vi "USBImageContinuousV1.5.vi"() -> ()   [LabVIEW 2017]
uses:
  <vilib>/Utility/file.llb/Write Delimited Spreadsheet (I64).vi
  atmcd32d.dll
panel:
  in  "Tab Control":T1(tab)
  out "Expected position on spectrometer (pixels):":dbl
  in  "Harmonic":dbl min=10.0 max=40.0
  out "l (nm)":dbl
  out "E (J)":dbl
  out "E (eV)":dbl
  out "Nearest Harmonic of 800nm":dbl
  out "Cursor Position (pixels)":dbl
  out "Distance to nearest harmonic of 800nm (pixels)":dbl
  in  "Grating:":u16(ring) items=["Shimadzu 30-006  "]
  in  "Laser:":u16(ring) items=["800nm  "]
  in  "Trigger":u32(ring) items=["Internal", "External"]
  in  "Exposure Time (secs)":sgl format="%.2f"
  out "Get Acquired Data":u32
  out "Start Acquisition":u32
  out "Detector X Pixels":i32
  out "Detector Y Pixels":i32
  out "Shut Down":u32
  out "Raw Image":i32[][](graph)
  out "Vertical Binned image":i32[](graph)
  out "Get Status":u32
  in  "Stop":bool
  in  "?":bool
  out "Camera Status:":bool
  out "Last Image Saved:":string
  in  "Calibration Date":u16(ring) items=["first calibration - 7/31", "7/31-current"]
  out "Calibration Date: indicator:":u16(ring) items=["first calibration - 7/31", "7/31-current"]
  out "Status":u32
  out "Camera outputs":T2
  out "Camera inputs":T3
  out "Wavelength Graph (nm)":cluster{"No prefix":dbl, i32}[](graph)
  out "Energy Graph (eV)":cluster{"eV":dbl, i32}[](graph)
  out "Harmonics Graph":cluster{"No prefix":dbl, i32}[](graph)
  # "Acquisition Mode: Single Scan\nReadout Mode: Full Resolution Image"
  # "Return values"
  # "XUV Spectrometer Control VI"
  # "Status"
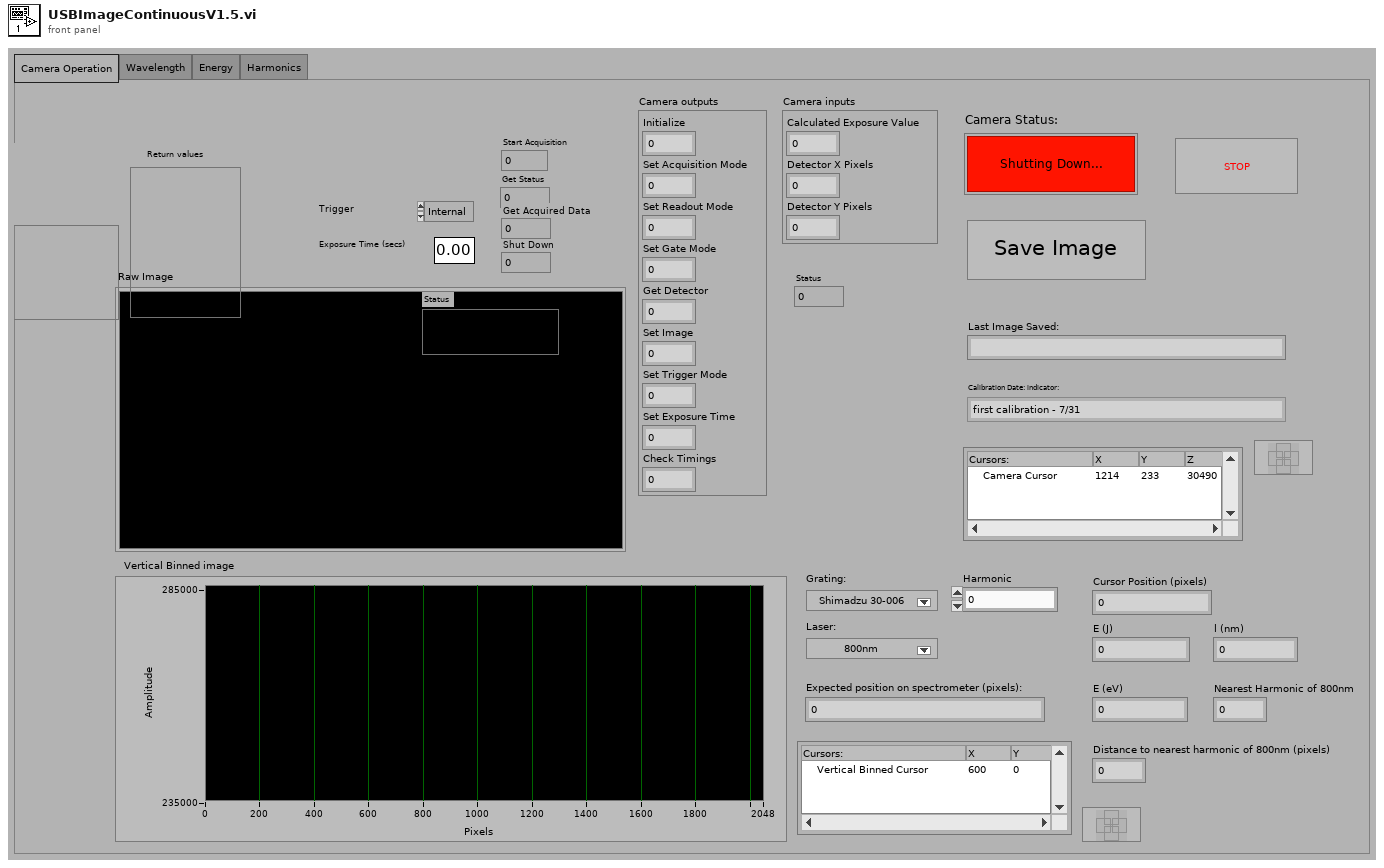
[diagram p1: front panel]
types:
  T1 = enum32{"Camera Operation", "Wavelength", "Energy", "Harmonics"}
  T2 = cluster{"Initialize":u32, "Set Acquisition Mode":u32, "Set Readout Mode":u32, "Set Gate Mode":u32, "Get Detector":u32, "Set Image":u32, "Set Trigger Mode":u32, "Set Exposure Time":u32, "Check Timings":u32}
  T3 = cluster{"Calculated Exposure Value":sgl, "Detector X Pixels":i32, "Detector Y Pixels":i32}
  T4 = cluster{"DRV_SUCCESS":i32, "to shutdown":bool, "to get acquired data":bool, "to start acquisition":bool}
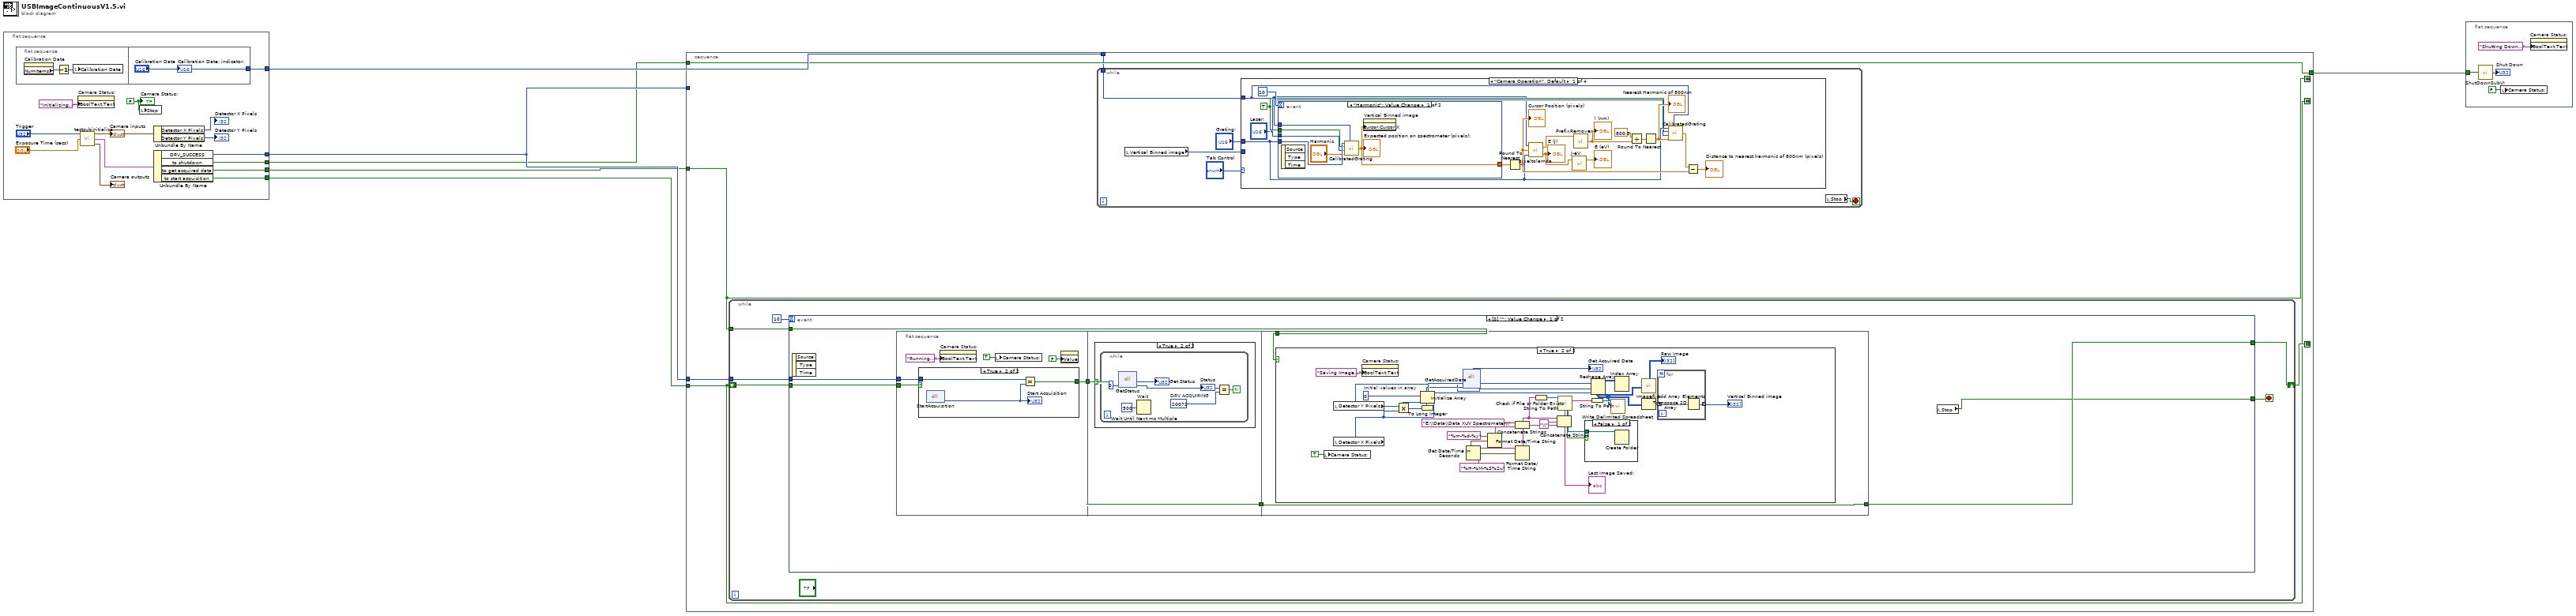
[diagram p0: block diagram]
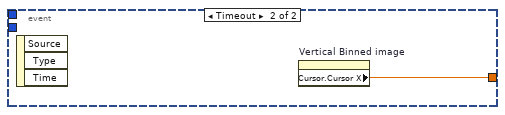
[diagram p2: hidden frame]
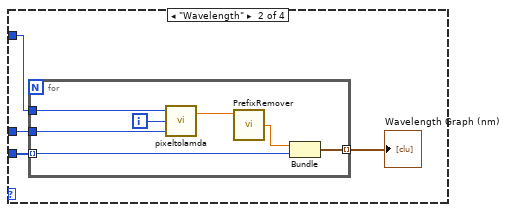
[diagram p3: hidden frame]
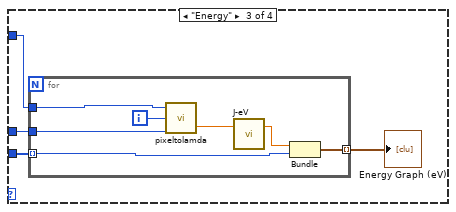
[diagram p4: hidden frame]
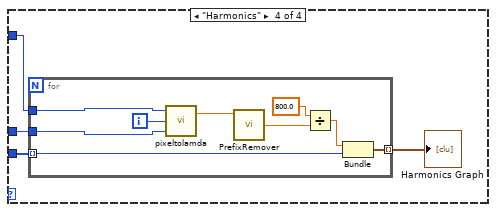
[diagram p5: hidden frame]
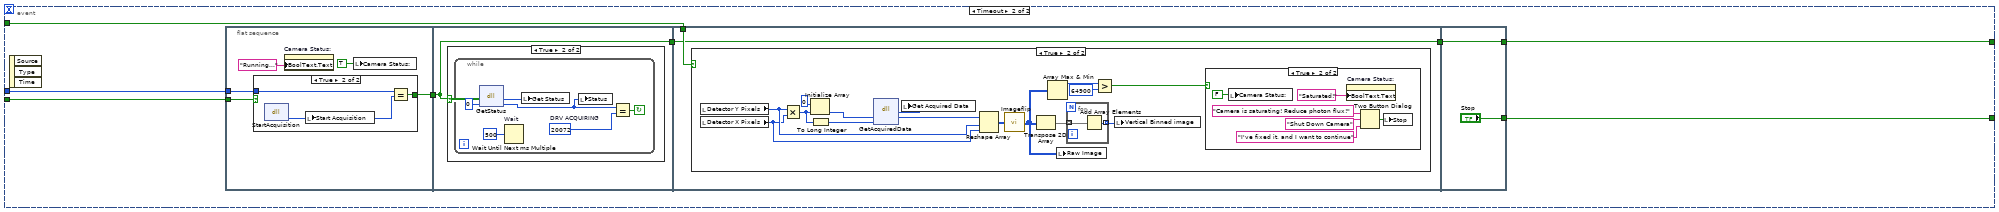
[diagram p10: hidden frame]
diagram:
  n1 = flat-sequence {
    tunnel: [w7] -> w6
    tunnel: [w8] -> w5
    tunnel: [w9] -> w4
    tunnel: [w10] -> w1
    tunnel: [w17] -> w2
    frame #0 {
      w18 = FALSE ("Camera Status:")
      n2 = flat-sequence {
        tunnel: ["Calibration Date"] -> w17
        frame #0 {
          n3 = property on="Calibration Date" class="Ring (strict)"() -> ("NumItems"=w22:u32)  [unwired: 2 in, 2 out]
          n4 = Decrement(x=w22) -> (x-1=w21:u32)
          n5 = local write "Calibration Date"(w21) -> ()
        }
        frame #1 {
          "Calibration Date: indicator:" <- "Calibration Date"
        }
      }
      n6 = property on="Camera Status:" class="Bool (strict)"("BoolText.Text"="Initializing..." ("String")) -> ()  [unwired: 2 in, 2 out]
      n7 = call "testsubinitialize.vi"("Exposure Time (secs)"="Exposure Time (secs)", "Trigger"="Trigger") -> ("Camera outputs"=→"Camera outputs":T2, "Camera status"=w14:T4, "Camera inputs"=w13:T3)  [unwired: 1 in]
      "Camera inputs" <- w13
      n8 = local write "Stop"(w18) -> ()
      n9 = Unbundle By Name(w13) -> ("Detector X Pixels"=→"Detector X Pixels":i32, "Detector Y Pixels"=→"Detector Y Pixels":i32)
      n10 = Unbundle By Name(w14) -> ("DRV_SUCCESS"=w7:i32, "to shutdown"=w10:bool, "to get acquired data"=w9:bool, "to start acquisition"=w8:bool)
      "Camera Status:" <- w18
    }
  }
  n11 = stacked-sequence {
    seq-local: [w27] -> [_]
    seq-local: [w28] -> [_]
    seq-local: [w26] -> [_]
    tunnel: w6 -> [_]
    tunnel: w6 -> [w29]
    tunnel: w5 -> [w27]
    tunnel: w4 -> [w26]
    tunnel: w1 -> [w25]
    tunnel: [w25] -> w3
    tunnel: w2 -> [w24]
    frame #0 {
      n12 = while {
        tunnel: w29 -> [w97]
        tunnel: w26 -> [w95]
        shift-right: [w96] -> w28
        shift-left: w27 -> [w98]
        stop <- w93 stop-if-true
        n13 = event shown="[0] \"\": Value Change" {
          selector: _ -> [_ _]
          dyn-events: _ -> [_ _]
          timeout: 10 -> [_ _]
          tunnel: w98 -> [w103 w160]
          tunnel: w97 -> [w102 w159]
          tunnel: [w101 w158] -> w96
          tunnel: w95 -> [w100 w157]
          tunnel: [w99 w156] -> w93
          event Value Change {
            n14 = event-data() -> ()  [unwired: 1 in, 3 out]
            n15 = flat-sequence {
              tunnel: w103 -> [w111]
              tunnel: w102 -> [w110]
              tunnel: [w109] -> w105
              tunnel: w105 -> [w116]
              tunnel: [w116] -> w104
              tunnel: [w124] -> w101
              tunnel: w104 -> [w124]
              tunnel: w100 -> [w123]
              frame #0 {
                n16 = case shown="True" w111 {
                  tunnel: [FALSE w114] -> w109
                  tunnel: w110 -> [_ w113]
                  frame False {
                  }
                  frame True {
                    n17 = dll-call lib="atmcd32d.dll" fn="StartAcquisition" label="Call Library Function start acquisition"() -> (w115:u32)  [unwired: 3 in, 2 out]
                    "Start Acquisition" <- w115
                    n18 = Equal?(x=w113, y=w115) -> (x = y?=w114:bool)
                  }
                }
                n19 = property on="Camera Status:" class="Bool (strict)"("BoolText.Text"="Running..." ("Boolean Text.Text")) -> ()  [unwired: 2 in, 2 out]
                n20 = local write "Camera Status:"(TRUE ("Camera Status:")) -> ()
                n21 = property class="Bool (strict)"("Value"=FALSE ("Take image")) -> ()  [unwired: 2 in, 2 out]
              }
              frame #1 {
                n22 = case shown="True" w116 {
                  frame False {
                  }
                  frame True {
                    n23 = while {
                      stop <- w120 continue-if-true
                      w119 = u16 20072  # DRV ACQUIRING
                      n24 = dll-call lib="atmcd32d.dll" fn="GetStatus" label="Call Library Function GetAcquisitionStatus"(u16 0) -> (→"Get Status":u32, w118:u32)  [unwired: 3 in, 2 out]
                      "Status" <- w118
                      n25 = Wait Until Next ms Multiple "Wait"(millisecond multiple=u32 500) -> ()  [unwired: 1 out]
                      n26 = Equal?(x=w118, y=w119) -> (x = y?=w120:bool)
                    }
                  }
                }
              }
              frame #2 {
                n27 = case shown="True" w123 {
                  frame False {
                  }
                  frame True {
                    w151 = 0  # Initial values in array
                    n28 = local write "Camera Status:"(TRUE ("Camera Status:")) -> ()
                    n29 = local read "Detector Y Pixels"() -> (w145:i32)
                    n30 = local read "Detector X Pixels"() -> (w144:i32)
                    n31 = property on="Camera Status:" class="Bool (strict)"("BoolText.Text"="Saving Image..." ("Boolean Text.Text")) -> ()  [unwired: 2 in, 2 out]
                    n32 = Multiply(x=w145, y=w144) -> (x*y=w147:i32)
                    n33 = To Long Integer(number=w147) -> (32bit integer=w148:i32)
                    n34 = Initialize Array "Initialize Array"(w151, w147) -> (w149:i32[])
                    n35 = dll-call lib="atmcd32d.dll" fn="GetAcquiredData" label="Call Library Function Get Acquired data"(w149, w148) -> (→"Get Acquired Data":u32, w146:i32[])  [unwired: 4 in, 2 out]
                    n36 = Get Date/Time In Seconds() -> (seconds since 1Jan1904=w141:timestamp)
                    n37 = Format Date/Time String(time format string (%c)="%m-%d-%y", seconds (now)=w141) -> (date/time string=w139:string)  [unwired: 1 in]
                    n38 = Concatenate Strings("E:\\Data\\Data XUV Spectrometer\\" ("string"), w139) -> (w142:string)
                    n39 = Format Date/Time String(time format string (%c)="%H-%M-%S%2u", seconds (now)=w141) -> (date/time string=w140:string)  [unwired: 1 in]
                    n40 = String To Path(string=w142) -> (path=w138:path)
                    n41 = Concatenate Strings(w142, "\\" ("string"), w140) -> (w143:string)
                    "Last Image Saved:" <- w143
                    n42 = call <vilib>:"Check if File or Folder Exists.vi"("path"=w138) -> ("file or folder exists?"=w136:bool, "dup path"=w137:path)  [unwired: 8 in, 1 out]
                    n43 = case shown="False" w136 {
                      tunnel: w137 -> [w154 _]
                      frame False {
                        n44 = Create Folder(path (use dialog)=w154) -> ()  [unwired: 2 in, 3 out]
                      }
                      frame True {
                      }
                    }
                    n45 = String To Path(string=w143) -> (path=w131:path)
                    n46 = Reshape Array(w146, w145, w144) -> (w126:i32[][])
                    n47 = call-poly <vilib>:"Write Delimited Spreadsheet.vi"("file path (dialog if empty)"=w131, "2D data"=w126) -> ()  [unwired: 12 in, 2 out]
                    n48 = Index Array(array=w126) -> ()  [unwired: 2 in, 1 out]
                    n49 = call "Imageflip.vi"("2D array"=w126) -> ("transposed array"=→"Raw Image":i32[][])
                    n50 = Transpose 2D Array(2D array=w126) -> (transposed array=w130:i32[][])
                    n51 = for {
                      tunnel: w130 -> [w153] mode=indexing
                      tunnel: [w152] -> w129 mode=indexing
                      n52 = Add Array Elements(numeric array=w153) -> (sum=w152:i32)
                    }
                    "Vertical Binned image" <- w129
                  }
                }
              }
            }
            n53 = local read "Stop"() -> (w99:bool)
          }
          event Timeout {
            n54 = event-data() -> ()  [unwired: 1 in, 3 out]
            n55 = flat-sequence {
              tunnel: w160 -> [w167]
              tunnel: w159 -> [w166]
              tunnel: [w165] -> w162
              tunnel: w162 -> [w172]
              tunnel: [w172] -> w161
              tunnel: w161 -> [w179]
              tunnel: w157 -> [w180]
              tunnel: [w179] -> w155
              tunnel: [w205] -> w158
              tunnel: w155 -> [w205]
              tunnel: ["Stop"] -> w156
              frame #0 {
                n56 = case shown="True" w167 {
                  tunnel: [FALSE w171] -> w165
                  tunnel: w166 -> [_ w170]
                  frame False {
                  }
                  frame True {
                    n57 = dll-call lib="atmcd32d.dll" fn="StartAcquisition" label="Call Library Function start acquisition"() -> (w169:u32)  [unwired: 3 in, 2 out]
                    n58 = local write "Start Acquisition"(w169) -> ()
                    n59 = Equal?(x=w170, y=w169) -> (x = y?=w171:bool)
                  }
                }
                n60 = property on="Camera Status:" class="Bool (strict)"("BoolText.Text"="Running..." ("Boolean Text.Text")) -> ()  [unwired: 2 in, 2 out]
                n61 = local write "Camera Status:"(TRUE ("Camera Status:")) -> ()
              }
              frame #1 {
                n62 = case shown="True" w172 {
                  frame False {
                  }
                  frame True {
                    n63 = while {
                      stop <- w176 continue-if-true
                      w175 = u16 20072  # DRV ACQUIRING
                      n64 = dll-call lib="atmcd32d.dll" fn="GetStatus" label="Call Library Function GetAcquisitionStatus"(u16 0) -> (w174:u32, w173:u32)  [unwired: 3 in, 2 out]
                      n65 = Wait Until Next ms Multiple "Wait"(millisecond multiple=u32 500) -> ()  [unwired: 1 out]
                      n66 = local write "Get Status"(w174) -> ()
                      n67 = local write "Status"(w173) -> ()
                      n68 = Equal?(x=w173, y=w175) -> (x = y?=w176:bool)
                    }
                  }
                }
              }
              frame #2 {
                n69 = case shown="True" w180 {
                  frame False {
                  }
                  frame True {
                    n70 = local read "Detector Y Pixels"() -> (w190:i32)
                    n71 = local read "Detector X Pixels"() -> (w183:i32)
                    n72 = Multiply(x=w190, y=w183) -> (x*y=w192:i32)
                    n73 = Initialize Array "Initialize Array"(0 ("Initial values in array"), w192) -> (w194:i32[])
                    n74 = To Long Integer(number=w192) -> (32bit integer=w193:i32)
                    n75 = dll-call lib="atmcd32d.dll" fn="GetAcquiredData" label="Call Library Function Get Acquired data"(w194, w193) -> (w188:u32, w191:i32[])  [unwired: 4 in, 2 out]
                    n76 = local write "Get Acquired Data"(w188) -> ()
                    n77 = Reshape Array(w191, w190, w183) -> (w181:i32[][])
                    n78 = call "Imageflip.vi"("2D array"=w181) -> ("transposed array"=w182:i32[][])
                    n79 = Transpose 2D Array(2D array=w182) -> (transposed array=w189:i32[][])
                    n80 = Array Max & Min(array=w182) -> (max value=w186:i32)  [unwired: 3 out]
                    n81 = local write "Raw Image"(w182) -> ()
                    n82 = for {
                      tunnel: w189 -> [w203] mode=indexing
                      tunnel: [w202] -> w187 mode=indexing
                      n83 = Add Array Elements(numeric array=w203) -> (sum=w202:i32)
                    }
                    n84 = Greater?(x=w186, y=64900) -> (0:w184:bool)
                    n85 = local write "Vertical Binned image"(w187) -> ()
                    n86 = case shown="True" w184 {
                      frame False {
                      }
                      frame True {
                        n87 = local write "Camera Status:"(FALSE ("Camera Status:")) -> ()
                        n88 = property on="Camera Status:" class="Bool (strict)"("BoolText.Text"="Saturated!" ("Boolean Text.Text")) -> ()  [unwired: 2 in, 2 out]
                        n89 = Two Button Dialog(message="Camera is saturating! Reduce photon flux!", 1:"I've fixed it, and I want to continue" ("message"), 2:"Shut Down Camera" ("T button name (\"OK\")")) -> (T button?=w197:bool)
                        n90 = local write "Stop"(w197) -> ()
                      }
                    }
                  }
                }
              }
              frame #3 {
              }
            }
          }
        }
      }
      n91 = while {
        tunnel: w24 -> [w30]
        stop <- w31 stop-if-true
        n92 = local read "Vertical Binned image"() -> (w33:i32[])
        n93 = case shown="\"Camera Operation\", Default" "Tab Control" {
          tunnel: w33 -> [_ w61 w72 w83]
          tunnel: "Grating:" -> [w38 w60 w71 w82]
          tunnel: w30 -> [w35 w58 w69 w80]
          frame "Camera Operation", Default {
            w37 = TRUE
            n94 = event shown="[0] \"Harmonic\": Value Change" {
              selector: _ -> [_ _]
              dyn-events: _ -> [_ _]
              timeout: 10 -> [_ _]
              tunnel: [w52 w57] -> w39
              tunnel: w38 -> [w56 _]
              tunnel: w37 -> [w55 _]
              tunnel: "Laser:" -> [w54 _]
              tunnel: w35 -> [w53 _]
              event "Harmonic": Value Change {
                n95 = event-data() -> ()  [unwired: 1 in, 3 out]
                n96 = call "CalibratedGrating.vi"("Grating:"=w56, "Subvi?"=w55, "Laser:"=w54, "Harmonic"="Harmonic", "Caibration Date"=w53) -> ("Position on spectrometer (pixels):"=w52:dbl)
                "Expected position on spectrometer (pixels):" <- w52
                n97 = property on="Vertical Binned image" class="WFGraph (strict)"("Cursor.Cursor X"=w52) -> ()  [unwired: 2 in, 2 out]
              }
              event Timeout {
                n98 = event-data() -> ()  [unwired: 1 in, 3 out]
                n99 = property on="Vertical Binned image" class="WFGraph (strict)"() -> ("Cursor.Cursor X"=w57:dbl)  [unwired: 2 in, 2 out]
              }
            }
            n100 = Round To Nearest(number=w39) -> (nearest integer value=w44:dbl)
            "Cursor Position (pixels)" <- w44
            n101 = call "pixeltolamda.vi"("Grating:"=w38, "Pixel Postion"=w44, "Caibration Date"=w35) -> ("E (J)"=w46:dbl, "lamda (m)"=w50:dbl)
            "E (J)" <- w46
            n102 = call "J-eV.vi"("J"=w46) -> ("eV"=→"E (eV)":dbl)  [unwired: 1 in, 1 out]
            n103 = call "PrefixRemover.vi"("Nano"=w50) -> ("No prefix"=w47:dbl)  [unwired: 3 in]
            "l (nm)" <- w47
            n104 = Divide(x=800.0, y=w47) -> (x/y=w49:dbl)
            n105 = Round To Nearest(number=w49) -> (nearest integer value=w43:dbl)
            "Nearest Harmonic of 800nm" <- w43
            n106 = call "CalibratedGrating.vi"("Grating:"=w38, "Subvi?"=w37, "Laser:"="Laser:", "Harmonic"=w43, "Caibration Date"=w35) -> ("Position on spectrometer (pixels):"=w42:dbl)
            n107 = Subtract(x=w42, y=w44) -> (x-y=→"Distance to nearest harmonic of 800nm (pixels)":dbl)
          }
          frame "Wavelength" {
            n108 = for {
              tunnel: w61 -> [w64] mode=indexing
              tunnel: w60 -> [w66]
              tunnel: [w63] -> w59 mode=indexing
              tunnel: w58 -> [w62]
              i -> [w65]
              n109 = call "pixeltolamda.vi"("Grating:"=w66, "Pixel Postion"=w65, "Caibration Date"=w62) -> ("lamda (m)"=w67:dbl)  [unwired: 1 out]
              n110 = call "PrefixRemover.vi"("Nano"=w67) -> ("No prefix"=w68:dbl)  [unwired: 3 in]
              n111 = Bundle("No prefix"=w68, w64) -> (w63:cluster{"No prefix":dbl, i32})  [unwired: 1 in]
            }
            "Wavelength Graph (nm)" <- w59
          }
          frame "Energy" {
            n112 = for {
              tunnel: w72 -> [w75] mode=indexing
              tunnel: w71 -> [w78]
              tunnel: [w74] -> w70 mode=indexing
              tunnel: w69 -> [w73]
              i -> [w79]
              n113 = call "pixeltolamda.vi"("Grating:"=w78, "Pixel Postion"=w79, "Caibration Date"=w73) -> ("E (J)"=w77:dbl)  [unwired: 1 out]
              n114 = call "J-eV.vi"("J"=w77) -> ("eV"=w76:dbl)  [unwired: 1 in, 1 out]
              n115 = Bundle("eV"=w76, w75) -> (w74:cluster{"eV":dbl, i32})  [unwired: 1 in]
            }
            "Energy Graph (eV)" <- w70
          }
          frame "Harmonics" {
            n116 = for {
              tunnel: w83 -> [w89] mode=indexing
              tunnel: w82 -> [w91]
              tunnel: [w88] -> w81 mode=indexing
              tunnel: w80 -> [w84]
              i -> [w90]
              n117 = call "pixeltolamda.vi"("Grating:"=w91, "Pixel Postion"=w90, "Caibration Date"=w84) -> ("lamda (m)"=w92:dbl)  [unwired: 1 out]
              n118 = call "PrefixRemover.vi"("Nano"=w92) -> ("No prefix"=w86:dbl)  [unwired: 3 in]
              n119 = Divide(x=800.0, y=w86) -> (x/y=w85:dbl)
              n120 = Bundle(w85, w89) -> (w88:cluster{dbl, i32})  [unwired: 1 in]
            }
            "Harmonics Graph" <- w81
          }
        }
        n121 = local read "Stop"() -> (w31:bool)
      }
    }
  }
  n122 = flat-sequence {
    tunnel: w3 -> [w207]
    frame #0 {
      n123 = call "ShutDownSubVI.vi"("shutdown"=w207) -> ("Shut Down"=→"Shut Down":u32)
      n124 = local write "Camera Status:"(FALSE ("Camera Status:")) -> ()
      n125 = property on="Camera Status:" class="Bool (strict)"("BoolText.Text"="Shutting Down..." ("Boolean Text.Text")) -> ()  [unwired: 2 in, 2 out]
    }
  }
